vi "Call Import ESI File.vi"(7 "Select a device profile or file path":path, 8 "error in":errorcluster, 9 "Import to RT target":bool, 10 "Import to host PC":bool, 11 "Target IP Address":string) -> (0 "error out":errorcluster, 3 "result out":string[][](array[string]))   [LabVIEW 2019, in "SEECD System Explorer.lvlib"]
uses:
  SEECD System Explorer.lvlib
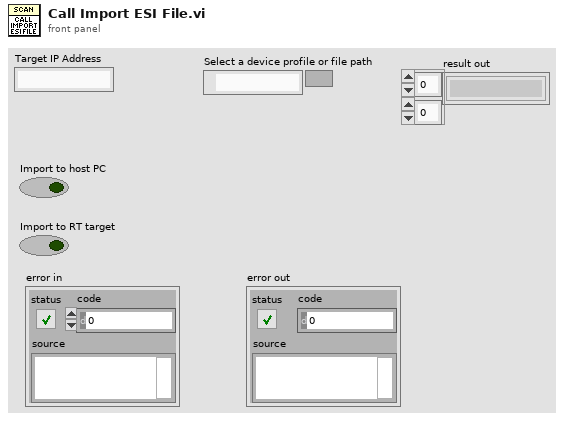
[diagram p1: front panel]
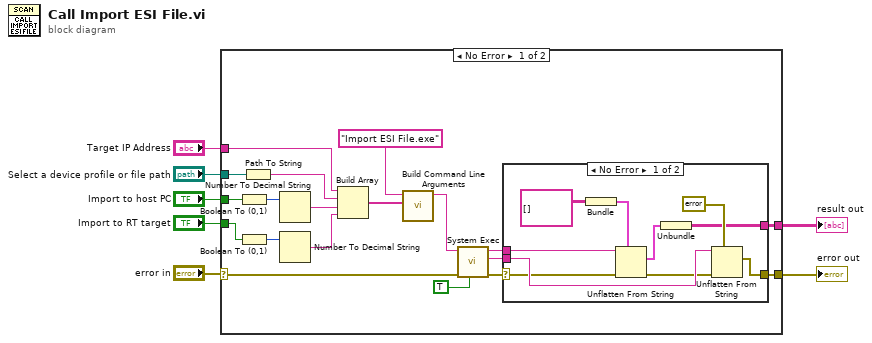
[diagram p0: block diagram]
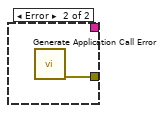
[diagram p2: hidden frame]
diagram:
  n1 = case shown="No Error" "error in" {
    selector: "error in" -> [w26 w38]
    tunnel: [w23 w38] -> w7
    tunnel: [w25 _] -> w5
    tunnel: "Import to RT target" -> [w14 _]
    tunnel: "Target IP Address" -> [w13 _]
    tunnel: "Select a device profile or file path" -> [w12 _]
    tunnel: "Import to host PC" -> [w9 _]
    frame No Error {
      n2 = Boolean To (0,1)(Boolean=w9) -> (0, 1=w10:i16)
      n3 = Boolean To (0,1)(Boolean=w14) -> (0, 1=w16:i16)
      n4 = Path To String(path=w12) -> (string=w11:string)
      n5 = Number To Decimal String(number=w10) -> (decimal integer string=w8:string)  [unwired: 1 in]
      n6 = Number To Decimal String(number=w16) -> (decimal integer string=w15:string)  [unwired: 1 in]
      n7 = Build Array(w13, w11, w8, w15) -> (w18:string[])
      n8 = call "Build Command Line Arguments.vi"("Arguments"=w18, "Executable File Name"="Import ESI File.exe" ("name or relative path")) -> ("Command Line"=w17:string)  [unwired: 9 in]
      n9 = call <vilib>:"System Exec.vi"("run minimized? (F)"=TRUE, "error in (no error)"=w26, "command line"=w17) -> ("error out"=w24:errorcluster, "standard error"=w21:string, "standard output"=w22:string)  [unwired: 5 in, 1 out]
      n10 = case shown="No Error" w24 {
        selector: w24 -> [w33 _]
        tunnel: [w29 _] -> w25
        tunnel: [w35 w37] -> w23
        tunnel: w22 -> [w32 _]
        tunnel: w21 -> [w34 _]
        frame No Error {
          n11 = Bundle("result out 2"=string[][] []) -> (w31:cluster{"result out 2":string[][]})  [unwired: 1 in]
          n12 = Unflatten From String(type=w31, binary string=w32, error in (no error)=w33) -> (value=w30:cluster{"result out 2":string[][]}, error out=w27:errorcluster)  [unwired: 2 in, 1 out]
          n13 = Unbundle(w30) -> ("result out 2"=w29:string[][])
          n14 = Unflatten From String(type=errorcluster {"status"=FALSE, "code"=0, "source"=""} ("error in (no error)"), binary string=w34, error in (no error)=w27) -> (value=w35:errorcluster)  [unwired: 2 in, 2 out]
        }
        frame Error {
          n15 = call "Generate Application Call Error.vi"() -> ("error out"=w37:errorcluster)  [unwired: 11 in]
        }
      }
    }
    frame Error {
    }
  }
  "error out" <- w7
  "result out" <- w5
